vi "Read Back Tunnel Internal TermRefs.vi"(8 "error in (no error)":errorcluster, 10 "element":string, 11 "CSM-Helper in":refnum<class "CSM-Helper.lvclass">) -> (0 "error out":errorcluster, 2 "Front Tunnels":T1, 3 "CSM-Helper out":refnum<class "CSM-Helper.lvclass">)   [LabVIEW 2020, in "CSM-Helper.lvclass"]
uses:
  CSM-Helper.lvclass
  CSM-Helper.lvclass/CSM-Helper.ctl
  Read Back Tunnels Refs.vi
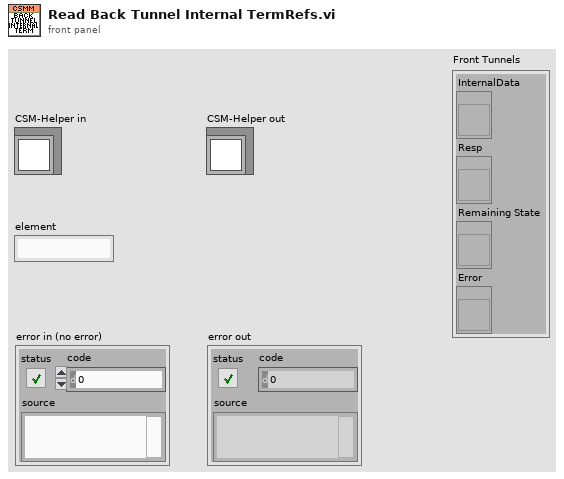
[diagram p1: front panel]
types:
  T1 = cluster{"InternalData":refnum<vi>, "Resp":refnum<vi>, "Remaining State":refnum<vi>, "Error":refnum<vi>}
  T2 = typedef "CSM-Helper.lvclass/_csmhelper_Back_Tunnels_Refs.ctl" = cluster{"InternalData":refnum<vi>, "Resp":refnum<vi>, "Remaining State":refnum<vi>, "Error":refnum<vi>}
  T3 = cluster{refnum<vi>, refnum<vi>, refnum<vi>, refnum<vi>}
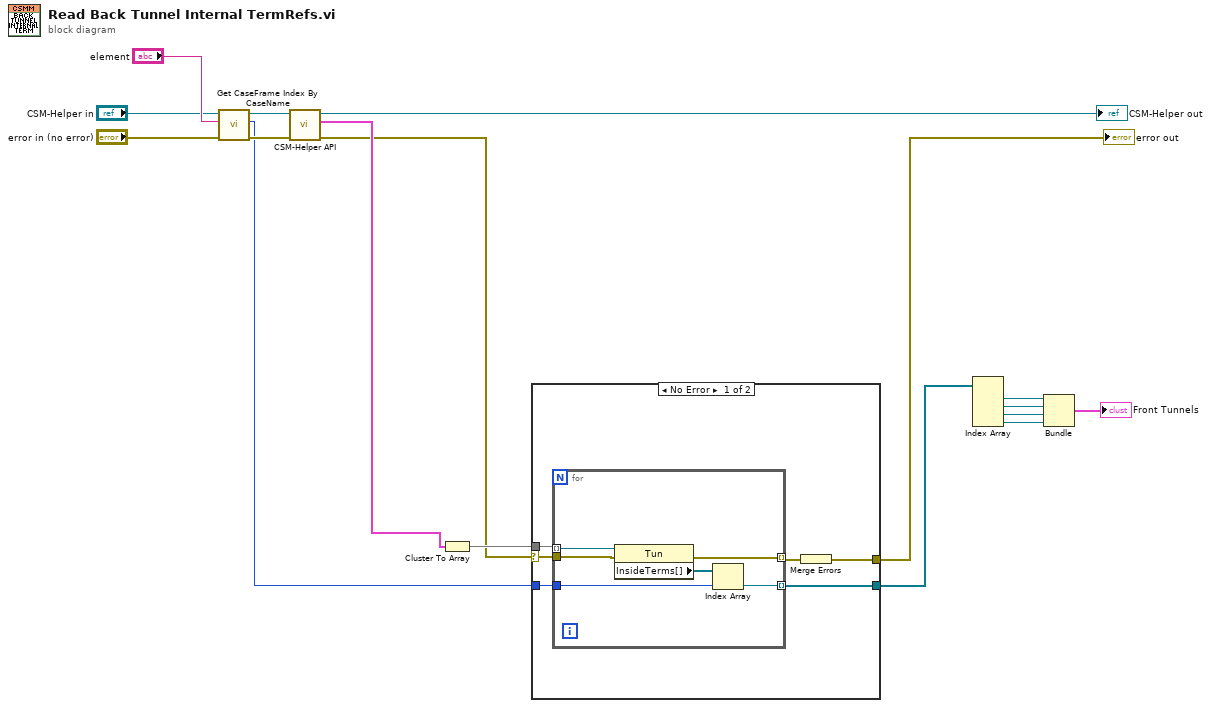
[diagram p0: block diagram]
diagram:
  n1 = call "Get CaseFrame Index By CaseName.vi"("error in (no error)"="error in (no error)", "CASE"="element", "CSM-Helper in"="CSM-Helper in") -> ("error out"=w17:errorcluster, "index"=w4:i32, "CSM-Helper out"=w15:refnum<class "CSM-Helper.lvclass">)  [unwired: 6 in]
  n2 = call-poly "CSM-Helper API.vi"("error in (no error)"=w17, "CSM-Helper in"=w15) -> ("error out"=w3:errorcluster, "Back Tunnels"=w5:T2, "CSM-Helper out"=→"CSM-Helper out":refnum<class "CSM-Helper.lvclass">)  [unwired: 7 in]
  n3 = Cluster To Array(cluster=w5) -> (array=w6:refnum<vi>[])
  n4 = case shown="No Error" w3 {
    selector: w3 -> [w19 w30]
    tunnel: [w23 _] -> w11
    tunnel: w6 -> [w21 _]
    tunnel: w4 -> [w20 _]
    tunnel: [w18 w30] -> w2
    frame No Error {
      n5 = for {
        tunnel: w20 -> [w28]
        tunnel: [w27] -> w23 mode=indexing
        tunnel: w21 -> [w26] mode=indexing
        tunnel: w19 -> [w25]
        tunnel: [w24] -> w22 mode=indexing
        n6 = property on="Property Node" class="Tun"(reference=w26, error in=w25) -> (error out=w24:errorcluster, "InsideTerms[]"=w29:refnum<vi>[])  [unwired: 1 out]
        n7 = Index Array(array=w29, index=w28) -> (element=w27:refnum<vi>)
      }
      n8 = Merge Errors(w22) -> (w18:errorcluster)
    }
    frame Error {
    }
  }
  "error out" <- w2
  n9 = Index Array(array=w11) -> (element #1=w10:refnum<vi>, element #2=w9:refnum<vi>, element #3=w8:refnum<vi>, element #4=w7:refnum<vi>)  [unwired: 4 in]
  n10 = Bundle(w10, w9, w8, w7) -> (→"Front Tunnels":T3)  [unwired: 1 in]
